vi "FillMeasFunc.vi"(8 "ErrorIn(No Error)":errorcluster caption="entrée d'erreur (pas d'erreur)", 9 "ActMeas":bool[](array[boolean]), 10 "MeasFunc":string[](array[string]), 11 "ListRef":refnum<vi>) -> (0 "sortie d'erreur":errorcluster, 3 "ActMeasOut":bool[](array[boolean]))   [LabVIEW 2019]
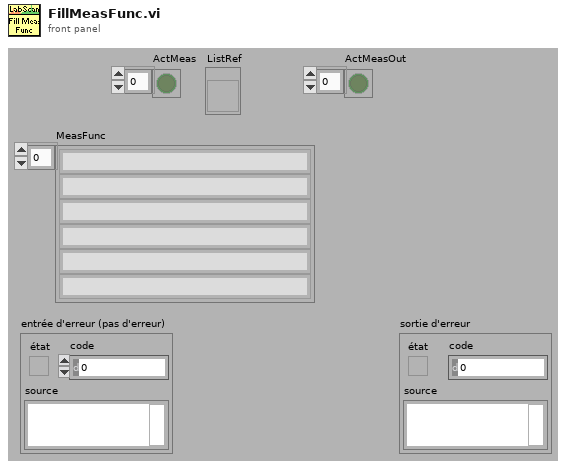
[diagram p1: front panel]
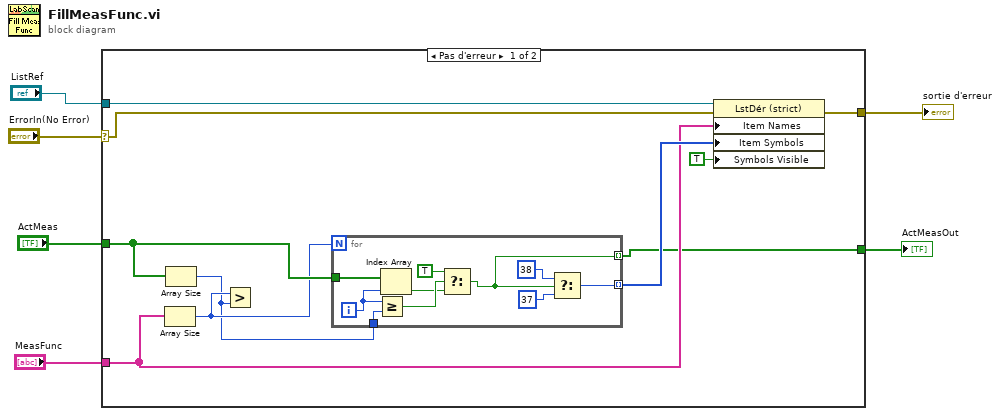
[diagram p0: block diagram]
diagram:
  n1 = case shown="Pas d'erreur" "ErrorIn(No Error)" {
    selector: "ErrorIn(No Error)" -> [w15 w28]
    tunnel: [w14 w28] -> w5
    tunnel: "MeasFunc" -> [w9 _]
    tunnel: "ListRef" -> [w16 _]
    tunnel: "ActMeas" -> [w13 w27]
    tunnel: [w8 w27] -> w1
    frame No Error {
      n2 = Array Size(array=w9) -> (size(s)=w12:i32)
      n3 = Array Size(array=w13) -> (size(s)=w11:i32)
      n4 = Greater?(x=w12, y=w11) -> ()  [unwired: 1 out]
      n5 = for {
        N: w12 -> [_]
        tunnel: w13 -> [w26]
        tunnel: w11 -> [w21]
        tunnel: [w18] -> w10 mode=indexing
        tunnel: [w17] -> w8 mode=indexing
        i -> [w25]
        n6 = Greater Or Equal?(x=w25, y=w21) -> (x >= y?=w24:bool)
        n7 = Index Array(array=w26, index=w25) -> (element=w23:bool)
        n8 = Select(t=TRUE ("cas vrai"), s=w24, f=w23) -> (s? t:f=w17:bool)
        n9 = Select(t=38, s=w17, f=37) -> (s? t:f=w18:i32)
      }
      n10 = property on="Nœud de propriété" class="LstDér (strict)"(reference=w16, error in=w15, "Item Names"=w9, "Item Symbols"=w10, "Symbols Visible"=TRUE ("Éléments visibles:Symboles visibles")) -> (error out=w14:errorcluster)  [unwired: 1 out]
    }
    frame Error {
    }
  }
  "sortie d'erreur" <- w5
  "ActMeasOut" <- w1
